vi "Propagate Parent State.vi"(8 "error in (no error)":errorcluster, 9 "Target in":refnum<class "State.lvclass">, 10 "Context in":refnum<class "Context.lvclass">, 11 "Source in":refnum<class "State.lvclass">) -> (0 "error out":errorcluster, 1 "Target out":refnum<class "State.lvclass">, 2 "Context out":refnum<class "Context.lvclass">, 3 "Source out":refnum<class "State.lvclass">)   [LabVIEW 2024, in "State.lvlib" / "State.lvclass"]
uses:
  State.lvclass
  Context/Context/Context.lvclass
  Container State/Container State.lvclass
  State.lvclass/State.ctl
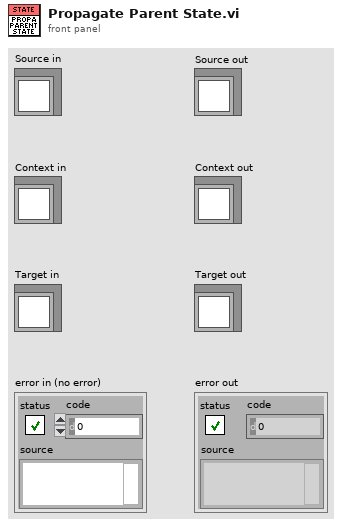
[diagram p1: front panel]
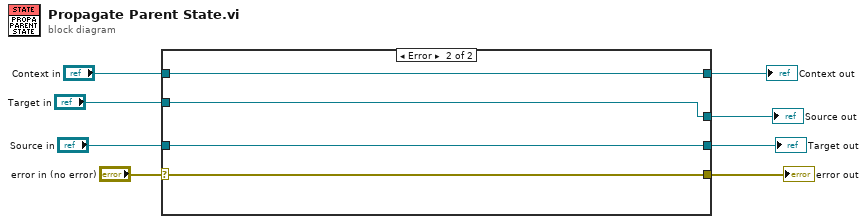
[diagram p0: block diagram]
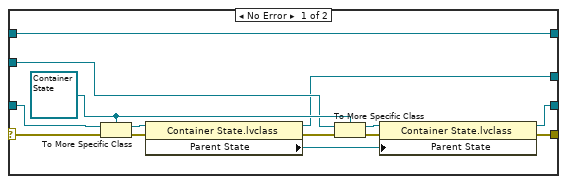
[diagram p2: hidden frame]
diagram:
  n1 = case shown="Error" "error in (no error)" {
    selector: "error in (no error)" -> [w20 w26]
    tunnel: [w13 w26] -> w7
    tunnel: [w12 w25] -> w5
    tunnel: "Source in" -> [w22 w25]
    tunnel: "Target in" -> [w17 w24]
    tunnel: [w10 w24] -> w3
    tunnel: [w9 w23] -> w2
    tunnel: "Context in" -> [w9 w23]
    frame No Error {
      w18 = refnum<class "Container State.lvclass"> refnum ("State.lvlib:Container State.lvclass")
      n2 = To More Specific Class(target class=w18, reference=w22, error in=w20) -> (specific class reference=w21:refnum<class "Container State.lvclass">, error out=w19:errorcluster)
      n3 = property class="Container State.lvclass"(reference=w21, error in=w19) -> (reference out=w10:refnum<class "Container State.lvclass">, error out=w16:errorcluster, "Parent State"=w11:refnum<class "State.lvclass">)
      n4 = To More Specific Class(target class=w18, reference=w17, error in=w16) -> (specific class reference=w15:refnum<class "Container State.lvclass">, error out=w14:errorcluster)
      n5 = property class="Container State.lvclass"(reference=w15, error in=w14, "Parent State"=w11) -> (reference out=w12:refnum<class "Container State.lvclass">, error out=w13:errorcluster)
    }
    frame Error {
    }
  }
  "error out" <- w7
  "Target out" <- w5
  "Source out" <- w3
  "Context out" <- w2
